vi "Z_ROI_compiler.vi"(0 "AOL_Globals":T2={"Imaging Protocol"=enum."AOL Z-Stack", "Number of POI"=0, "Number of Miniscans"=0, "Number of Trials"=0, "Number of Cycles "=0, "# Averaged Frames"=0, "Laser power (%)"=0, "Pockels (V)"=0.0, "Acquisition Length (sec)"=0.0, "Fill time (us)"=0.0, "POI Dwell time (us)"=0.0, "Miniscan Dwell time per pixel (us)"=0.0, "PMT 1"=0.0, "PMT 2"=0.0, "Back Apperture (mA)"=200.0, "Frame Size"=0, "Center Frequency"=0.0, "Field of View (um)"=175.0, "Field of View (norm)"=0.0, "DwellTime (us)"=0.0, "Ref Dwell Time (us)"=0.0, "Wavelength (nm)"=0.0, "Zoom"=0.0, "AOL Z"=0.0, "AOL Mode"=enum."Raster", "GridXY"=0.0, "GridZ"=0.0, "TriggerPeriod (sec)"=0.0, "Number of Pixels in Miniscan"=0, "Experiment folder path"=path "", "X centre"=0.0, "Y centre"=0.0, "Angle (degrees)"=0.0, "Angle Xs (degrees)"=0.0, "Angle Ys (degrees)"=0.0, "Plane Mode"=0, "Threshold"=[], "Regenerate Chirps"=FALSE, "Rectangle ROI length (pixels)"=0, "Rectangle ROI height (pixels)"=0, "AOD fill"=4900, "StartupDelay"=0, "Samples Wait after Trigger"=5080, "Slip Cycle"=600000, "Add Cycle"=TRUE, "Functional Mode"=enum."Point", "Z Start"=0.0, "Z Stop"=0.0, "# Planes"=0, "Total Pixels"=0, "Variable Miniscan Pixels"=[], "Use Variable Length"=FALSE, "Use Variable Resolution"=FALSE, "Laser power (%) at Z Start"=0, "Laser power (%) at Z Stop"=0, "Ref Z Step"=0} {"Angle Ys (degrees)" format="%#.6g"; "Angle Xs (degrees)" format="%#.6g"; "Plane Mode" items=["XY Plane", "XZ Plane", "YZ Plane", "arbitraryplane"]; "Frame Size" items=["100X100"=100, "128X128"=128, "200X200"=200, "256X256"=256, "512X512"=512, "1024x1024"=1024, "2048x2048"=2048]; "Back Apperture (mA)" format="%#.6g"; "Pockels (V)" format="%#.6g"; "PMT 2" format="%#.6g"; "PMT 1" format="%#.6g"; "Angle (degrees)" format="%#.6g"; "POI Dwell time (us)" format="%#.6g"}, 1 "dISABLE":bool=TRUE, 5 "Acquired z-plane index / volume index":i32, 11 "error in (no error)":errorcluster) -> (2 "Laser(V)":dbl[](array[numeric]), 3 "Zoom":dbl[](array[numeric]), 4 "Cycle time (us)":dbl, 6 "ROI Coordinates (broken down to miniscans)":T8, 10 "AOL_Globals":T2={"Imaging Protocol"=enum."AOL Z-Stack", "Number of POI"=0, "Number of Miniscans"=0, "Number of Trials"=0, "Number of Cycles "=0, "# Averaged Frames"=0, "Laser power (%)"=0, "Pockels (V)"=0.0, "Acquisition Length (sec)"=0.0, "Fill time (us)"=0.0, "POI Dwell time (us)"=0.0, "Miniscan Dwell time per pixel (us)"=0.0, "PMT 1"=0.0, "PMT 2"=0.0, "Back Apperture (mA)"=200.0, "Frame Size"=0, "Center Frequency"=0.0, "Field of View (um)"=175.0, "Field of View (norm)"=0.0, "DwellTime (us)"=0.0, "Ref Dwell Time (us)"=0.0, "Wavelength (nm)"=0.0, "Zoom"=0.0, "AOL Z"=0.0, "AOL Mode"=enum."Raster", "GridXY"=0.0, "GridZ"=0.0, "TriggerPeriod (sec)"=0.0, "Number of Pixels in Miniscan"=0, "Experiment folder path"=path "", "X centre"=0.0, "Y centre"=0.0, "Angle (degrees)"=0.0, "Angle Xs (degrees)"=0.0, "Angle Ys (degrees)"=0.0, "Plane Mode"=0, "Threshold"=[], "Regenerate Chirps"=FALSE, "Rectangle ROI length (pixels)"=0, "Rectangle ROI height (pixels)"=0, "AOD fill"=4900, "StartupDelay"=0, "Samples Wait after Trigger"=5080, "Slip Cycle"=600000, "Add Cycle"=TRUE, "Functional Mode"=enum."Point", "Z Start"=0.0, "Z Stop"=0.0, "# Planes"=0, "Total Pixels"=0, "Variable Miniscan Pixels"=[], "Use Variable Length"=FALSE, "Use Variable Resolution"=FALSE, "Laser power (%) at Z Start"=0, "Laser power (%) at Z Stop"=0, "Ref Z Step"=0} {"Angle Ys (degrees)" format="%#.6g"; "Angle Xs (degrees)" format="%#.6g"; "Plane Mode" items=["XY Plane", "XZ Plane", "YZ Plane", "arbitraryplane"]; "Frame Size" items=["100X100"=100, "128X128"=128, "200X200"=200, "256X256"=256, "512X512"=512, "1024x1024"=1024, "2048x2048"=2048]; "Back Apperture (mA)" format="%#.6g"; "Pockels (V)" format="%#.6g"; "PMT 2" format="%#.6g"; "PMT 1" format="%#.6g"; "Angle (degrees)" format="%#.6g"; "POI Dwell time (us)" format="%#.6g"}, 12 "NO ROI AVAILABLE!!!":bool, 13 "ROI Attributes (broken down to miniscans)":T1[](array[typedef]) {"Apparent Frame Size" format="%#_6f"; "Original FOV (um)" format="%#_6f"; "Pixels per miniscan" format="%#_6f"; "Dwell Time per pixel" format="%#_6f"; "Resolution" format="%#_6f"; "ROI group ID" format="%#_6f"; "Laser Power (%)" format="%#_6f"; "Zoom" format="%#_6f"; "Frame Size" format="%#_6f"; "Number of lines" format="%#_6f"; "Composite ID" format="%#_6f"; "Angle (deg)" format="%#_6f"; "ROI Time (ns)" format="%#_6f"; "ROI ID" format="%#_6f"; "Pixels in ROI" format="%#_6f"; "ROI index" format="%#_6f"; "Z stop" format="%#_6f"; "Y stop" format="%#_6f"; "X stop" format="%#_6f"; "Z start" format="%#_6f"; "X start" format="%#_6f"; "Y start" format="%#_6f"}, 15 "error out":errorcluster)   [LabVIEW 2020]
uses:
  Typedefs/ROI XY coordinates cluster.ctl
  Typedefs/Controls/AOL_Globals.ctl
  Typedefs/Imaging Protocols enum.ctl
  Typedefs/Frame Size.ctl
  Typedefs/AOL modes.ctl
  Typedefs/Plane Mode.ctl
  Typedefs/Functional Mode.ctl
  User Interface/Visualisation/Functional Imaging Viewer/Typedefs/ROI parameters data type.ctl
  User Interface/Visualisation/Functional Imaging Viewer/SubVIs/Experiment header interface/Typedefs/Header file sections.ctl
  User Interface/Visualisation/Functional Imaging Viewer/SubVIs/Experiment header interface/Typedefs/Header file actions.ctl
  User Interface/Visualisation/Functional Imaging Viewer/SubVIs/Experiment header interface/Typedefs/Save-Load-Save as-Load last enum.ctl
  User Interface/Visualisation/Functional Imaging Viewer/SubVIs/Experiment header interface/Typedefs/Header file type enum.ctl
panel:
  # "PRE-ALLOCATED CLONE RE-ENTRANT"
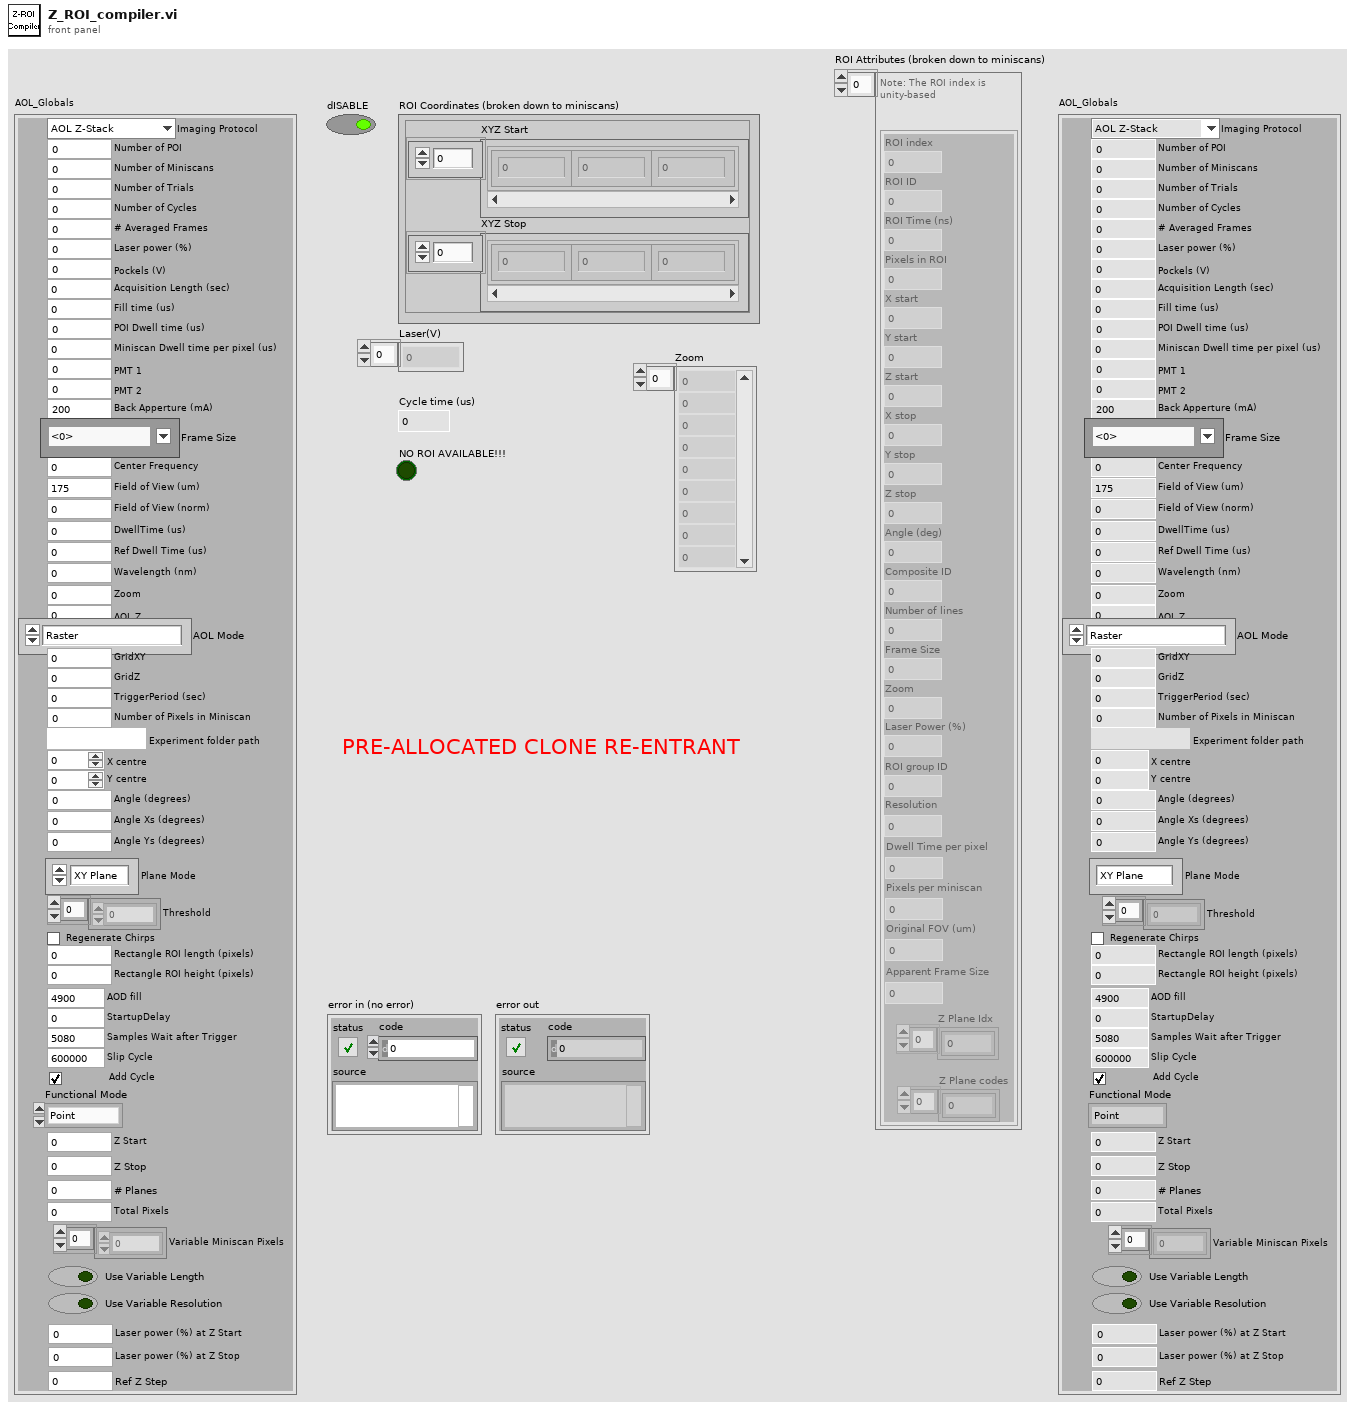
[diagram p1: front panel]
types:
  T1 = typedef "ROI parameters data type.ctl" = cluster{"ROI index":dbl, "ROI ID":dbl, "ROI Time (ns)":dbl, "Pixels in ROI":dbl, "X start":dbl, "Y start":dbl, "Z start":dbl, "X stop":dbl, "Y stop":dbl, "Z stop":dbl, "Angle (deg)":dbl, "Composite ID":dbl, "Number of lines":dbl, "Frame Size":dbl, "Zoom":dbl, "Laser Power (%)":dbl, "ROI group ID":dbl, "Resolution":dbl, "Dwell Time per pixel":dbl, "Pixels per miniscan":dbl, "Original FOV (um)":dbl, "Apparent Frame Size":dbl, "Z Plane Idx":i32[], "Z Plane codes":i32[]}
  T2 = typedef "AOL_Globals.ctl" = cluster{"Imaging Protocol":T3, "Number of POI":u16, "Number of Miniscans":u16, "Number of Trials":u16, "Number of Cycles ":u64, "# Averaged Frames":u16, "Laser power (%)":u8, "Pockels (V)":dbl, "Acquisition Length (sec)":dbl, "Fill time (us)":dbl, "POI Dwell time (us)":dbl, "Miniscan Dwell time per pixel (us)":dbl, "PMT 1":dbl, "PMT 2":dbl, "Back Apperture (mA)":dbl, "Frame Size":T4, "Center Frequency":dbl, "Field of View (um)":dbl, "Field of View (norm)":dbl, "DwellTime (us)":dbl, "Ref Dwell Time (us)":dbl, "Wavelength (nm)":dbl, "Zoom":dbl, "AOL Z":dbl, "AOL Mode":T5, "GridXY":dbl, "GridZ":dbl, "TriggerPeriod (sec)":dbl, "Number of Pixels in Miniscan":u16, "Experiment folder path":path, "X centre":dbl, "Y centre":dbl, "Angle (degrees)":dbl, "Angle Xs (degrees)":dbl, "Angle Ys (degrees)":dbl, "Plane Mode":T6, "Threshold":u16[], "Regenerate Chirps":bool, "Rectangle ROI length (pixels)":u16, "Rectangle ROI height (pixels)":u16, "AOD fill":u16, "StartupDelay":i32, "Samples Wait after Trigger":u16, "Slip Cycle":u32, "Add Cycle":bool, "Functional Mode":T7, "Z Start":dbl, "Z Stop":dbl, "# Planes":i32, "Total Pixels":i32, "Variable Miniscan Pixels":u16[], "Use Variable Length":bool, "Use Variable Resolution":bool, "Laser power (%) at Z Start":u8, "Laser power (%) at Z Stop":u8, "Ref Z Step":i8}
  T3 = typedef "Imaging Protocols enum.ctl" = enum16{"AOL Z-Stack", "Motor Z Stack", "Parameter Sweep", "Functional Acquisition", "Single Plane Acquisition", "Volume Acquisition", "Live Imaging", "Live Plane Imaging", "Live Volume Imaging"}
  T4 = typedef "Frame Size.ctl" = u16
  T5 = typedef "AOL modes.ctl" = enum16{"Raster", "Structural", "Pointing", "Mini Scan", "Alignment"}
  T6 = typedef "Plane Mode.ctl" = u16
  T7 = typedef "Functional Mode.ctl" = enum16{"Point", "Line", "Patch", "Plane", "Volume"}
  T8 = typedef "ROI XY coordinates cluster.ctl" = cluster{"XYZ Start":cluster{"X":sgl, "Y":sgl, "Z":sgl}[], "XYZ Stop":cluster{"X":sgl, "Y":sgl, "Z":sgl}[]}
  T9 = typedef "Header file actions.ctl" = enum16{"Create", "Open", "Read All", "Read Section", "Write All", "Write Section", "Close"}
  T10 = typedef "Header file sections.ctl" = enum16{"ALL SECTIONS", "LOGIN", "GLOBAL PARAMETERS", "CALIBRATION DATA", "IMAGING MODES", "TIME SERIES", "MOTOR Z-STACK", "AOL Z-STACK", "FUNCTIONAL IMAGING", "VOLUME IMAGING", "MOVEMENT CORRECTION", "CALIBRATION", "STATISTICS", "BIOLOGY INFORMATION"}
  T11 = typedef "Header file type enum.ctl" = enum16{"All parameters", "Params for funct acq w ROI or mscn", "Params for funct acq w rectangles", "Live imaging header parameters", "AOL Parameters"}
  T12 = typedef "Save-Load-Save as-Load last enum.ctl" = enum16{"Save file", "Save file as", "Load file", "Load last file"}
  T13 = typedef "Header parameters cluster-ALL.ctl" = cluster{"LOGIN":T14, "GLOBAL PARAMETERS":T15, "IMAGING MODES":T17, "TIME SERIES":T18, "MOTOR Z-STACK ":T20, "AOL Z-STACK":T21, "FUNCTIONAL IMAGING":T22, "VOLUME IMAGING":T22, "MOVEMENT CORRECTION":T23, "CALIBRATION":T25, "STATISTICS":T26, "BIOLOGY INFORMATION":T27, "Calibration Data":T28}
  T14 = typedef "Header params -Login.ctl" = cluster{"User":string, "Profile":string, "Software Version":string, "Experiment Date Time":timestamp}
  T15 = typedef "Header params-Global Parameters.ctl" = cluster{"MicroscopeID":string, "Microscope Type":string, "Objective":string, "Field of View (um)":dbl, "Fill time (us)":dbl, "Experiment Type":T16, "Stimuli Trigger":bool, "Speed Logging":bool}
  T16 = typedef "Experiment Type.ctl" = enum16{"In vivo", "In vitro", "Testing", "Calibration", "Other"}
  T17 = typedef "Header params-Imaging Modes.ctl" = cluster{"Time Series":bool, "Motor Zstack":bool, "AOL Zstack":bool, "Functional Imaging":bool, "Volume Imaging":bool}
  T18 = typedef "Header params-Time Series.ctl" = cluster{"Basic Image meta data":T19, "AOL z":dbl}
  T19 = typedef "Header params-Basic image meta data.ctl" = cluster{"Wavelength (nm)":dbl, "# averaged frames":dbl, "laser power (%)":dbl, "Pockels":dbl, "pixel dwell time (us)":dbl, "pmt 1":dbl, "pmt 2":dbl, "back apperture":dbl, "zoom":dbl, "field of view":dbl, "Frame Size":T4, "AOL x centre":dbl, "AOL y centre":dbl, "Stage x position":dbl, "Stage y position":dbl, "Stage z position":dbl}
  T20 = typedef "Header params-Motor Z-stack.ctl" = cluster{"Hdr Basic Image meta data":T19, "Z Start":dbl, "Z Stop":dbl, "No of Planes":i32, "Laser Power (%) at Z Start":dbl, "Laser Power (%) at Z Stop":dbl}
  T21 = typedef "Header params-AOL Z-stack.ctl" = cluster{"Hdr Basic Image meta data":T19, "Z Start":dbl, "Z Stop":dbl, "No of Planes":i32, "Laser Power (%) at Z Start":dbl, "Laser Power (%) at Z Stop":dbl}
  T22 = typedef "Header params-Functional Imaging.ctl" = cluster{"Functional Mode":T7, "Variable Length":bool, "Variable Resolution":bool, "Pockels Modulation":bool, "Stimuli Trigger":bool, "Cool down enabled":bool, "AOL Mode":T5, "Plane Mode":T6, "Miniscan Dwell time per pixel (us)":dbl, "poi dwell time":dbl, "Number of trials":dbl, "Number of cycles":dbl, "Number of pois":dbl, "Number of miniscans":dbl, "Number of pixels in miniscan":dbl, "Rectangle ROI length":dbl, "Rectangle ROI height":dbl, "Frame rate (fps)":dbl, "Acquisition Length":dbl, "video length (sec)":dbl, "Stimuli delay (sec)":dbl, "Cool down time (sec)":dbl, "Basic Image meta data":T19, "Z Start (um)":dbl, "Z Stop (um)":dbl}
  T23 = typedef "Header params-Movement correction.ctl" = cluster{"Movement Correction":bool, "Axial Reference":bool, "Reference Source":T24, "Full Frame Size":dbl, "Reference Field of View":dbl, "Reference Zoom":dbl, "Reference dwell time (us)":dbl, "Reference X Pixels":dbl, "Reference Y Pixels":dbl, "Number of Z lines":dbl, "Size of Z pixels":dbl, "Axial Pixels":dbl, "Ignore Z lines":dbl, "Reference Scan Cycles":dbl, "Reference Threshold XY":dbl, "Reference Threshold Z":dbl, "Reference Average XY":dbl, "Reference Average Z":dbl, "Proportional Scale":dbl, "Integral Scale":dbl, "Proportional Scale Z":dbl, "Integral Scale Z":dbl, "Diff Threshold":dbl, "Diff Threshold Z":dbl, "Sliding Average":bool, "Reference count reset enabled":bool, "Scan Interval (ms)":dbl, "Ref Plot Refresh Rate (ms)":dbl}
  T24 = typedef "Reference source.ctl" = enum16{"Green channel", "Red channel"}
  T25 = typedef "Header params-Calibration Setup.ctl" = cluster{"Pockels Calibration File":path, "Calibration_ini file":path, "Setup_ini file":path}
  T26 = typedef "Header params-statistics.ctl" = cluster{"Z-stack duration (sec)":dbl, "Number of acquired data-points":dbl, "Acquisition time (ms)":dbl, "Number of acquired frames":dbl, "Intertrial times":dbl[]}
  T27 = typedef "Biology Information.ctl" = cluster{"Animal Code or Name":string, "Animal DoB":string, "Animal Age":string, "Animal Sex":string, "Animal Weight":string, "Date of Injection":string, "Date of Implant":string, "Site of Injection":string, "Animal Ear Notch":string, "AAV constructs":string, "Genetic background":string, "Optical reporter":string, "Region of brain imaged":string, "Other \ncomments":string}
  T28 = typedef "Header params-calibration data.ctl" = cluster{"Objective Name":string, "Calibration Wavelength":dbl, "Sum X":dbl, "Sum Y":dbl, "Diff X":dbl, "Diff Y":dbl, "Distortion Correction":dbl, " Z norm to um Scaling":dbl, " X norm to um Scaling":dbl}
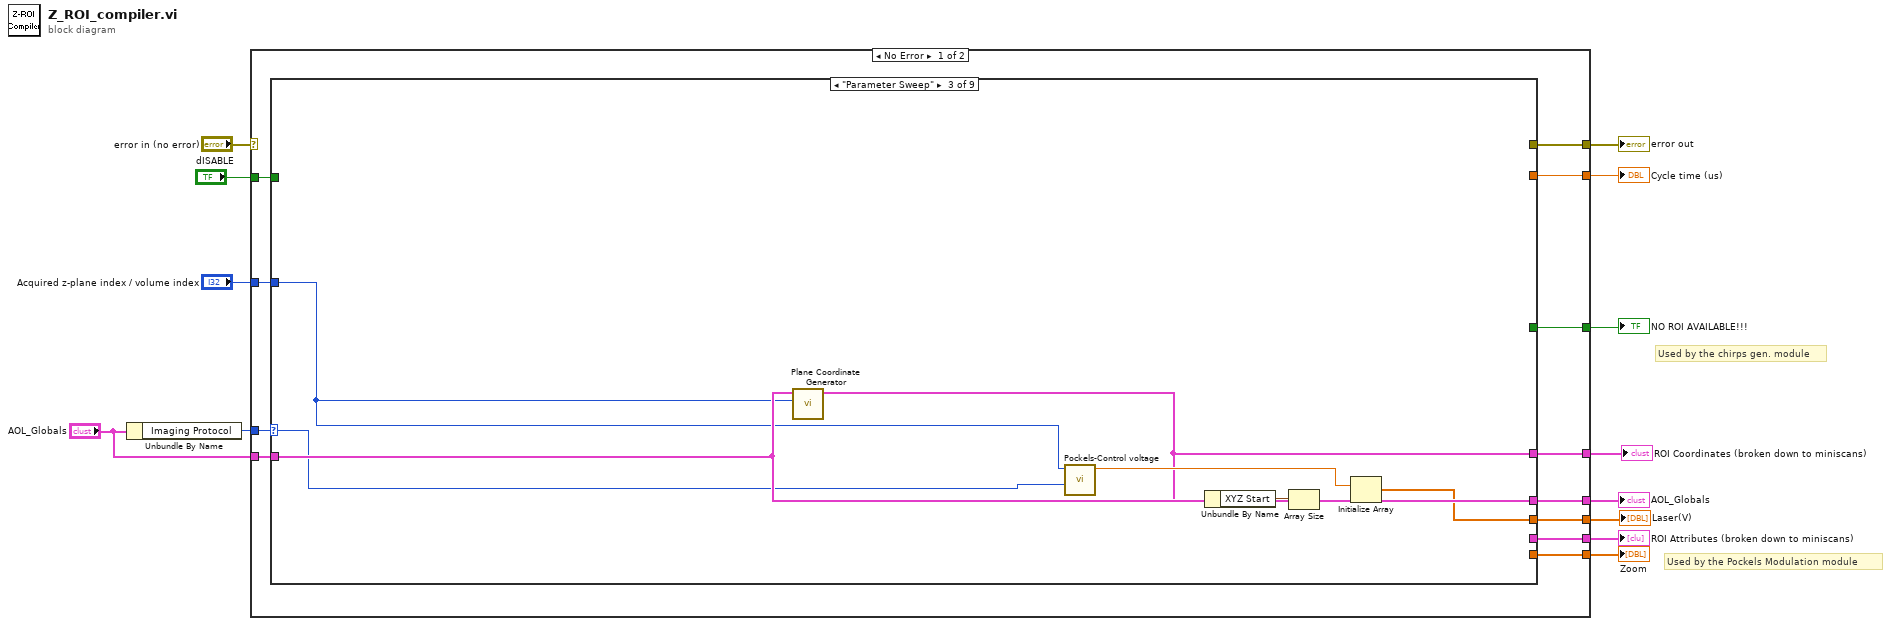
[diagram p0: block diagram]
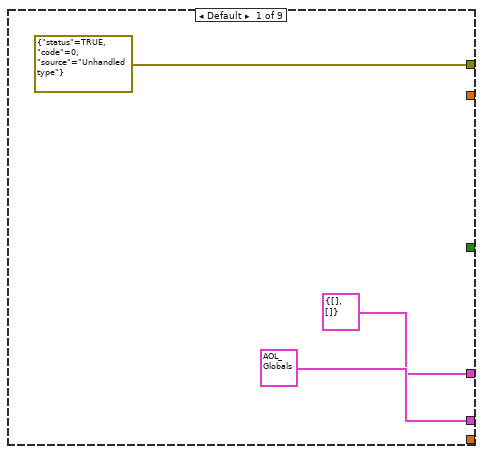
[diagram p2: hidden frame]
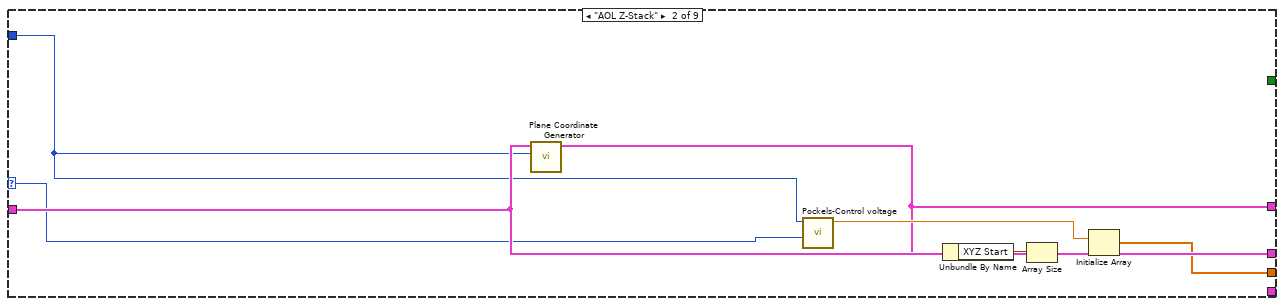
[diagram p3: hidden frame]
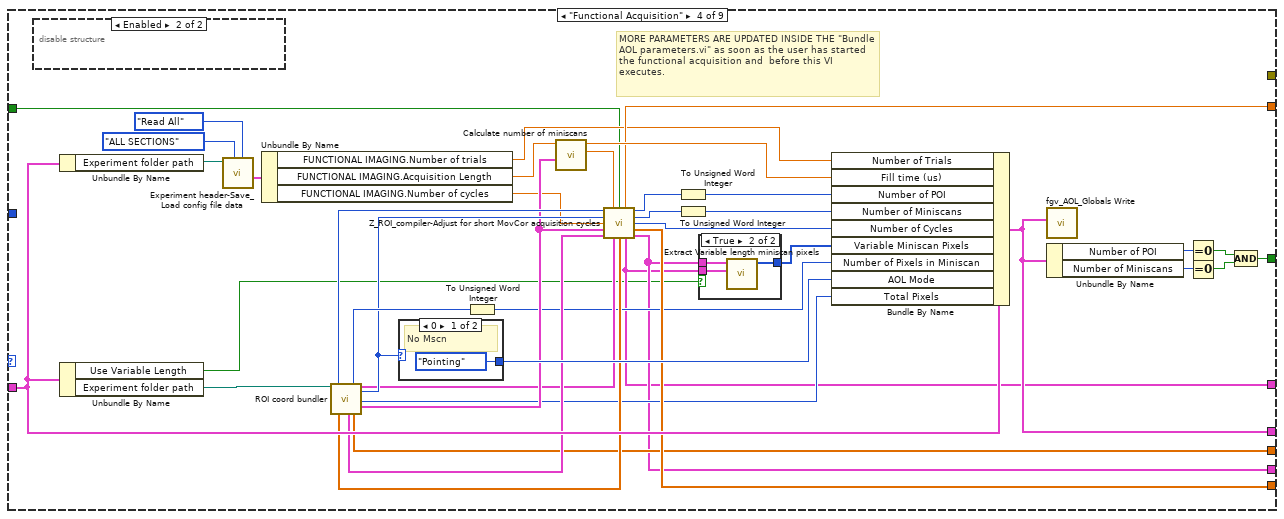
[diagram p4: hidden frame]
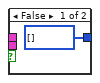
[diagram p5: hidden frame]
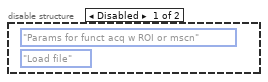
[diagram p6: hidden frame]
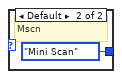
[diagram p7: hidden frame]
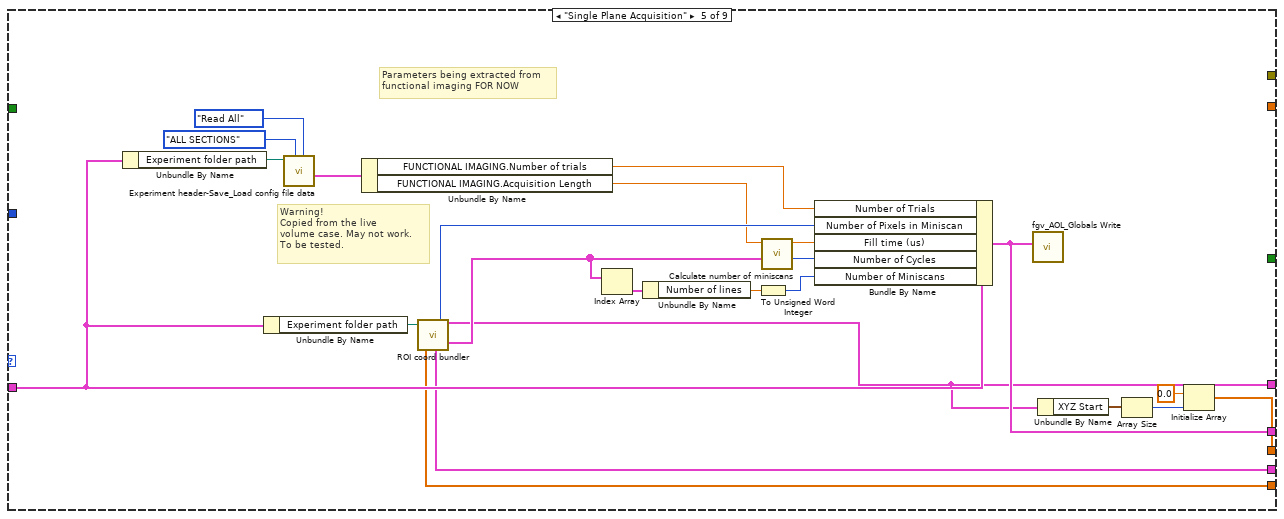
[diagram p8: hidden frame]
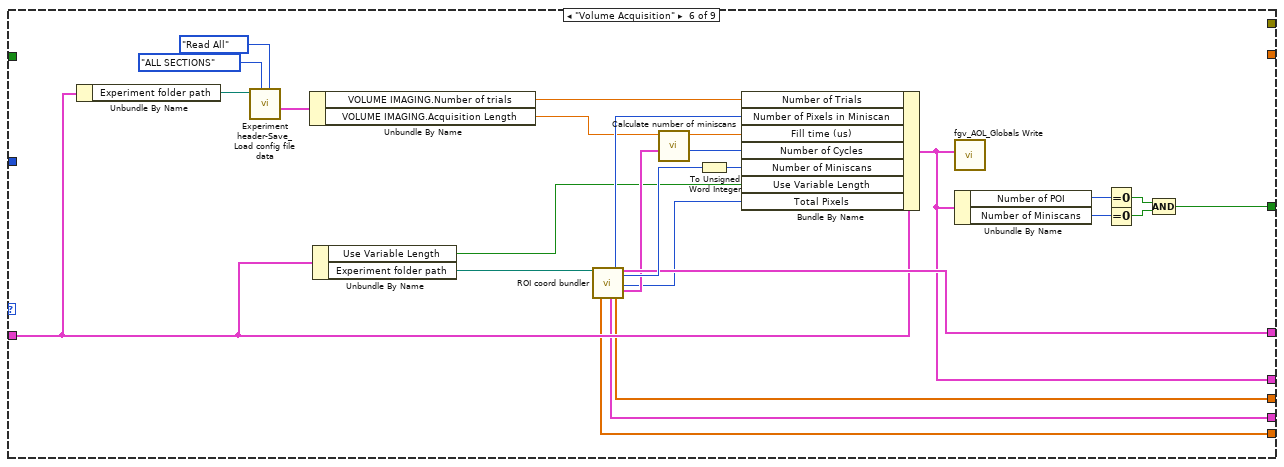
[diagram p9: hidden frame]
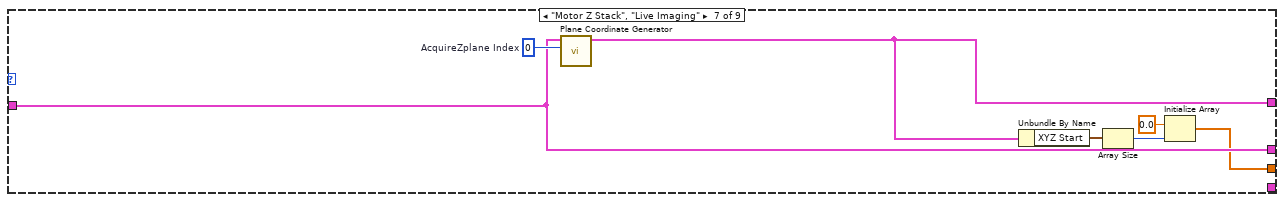
[diagram p10: hidden frame]
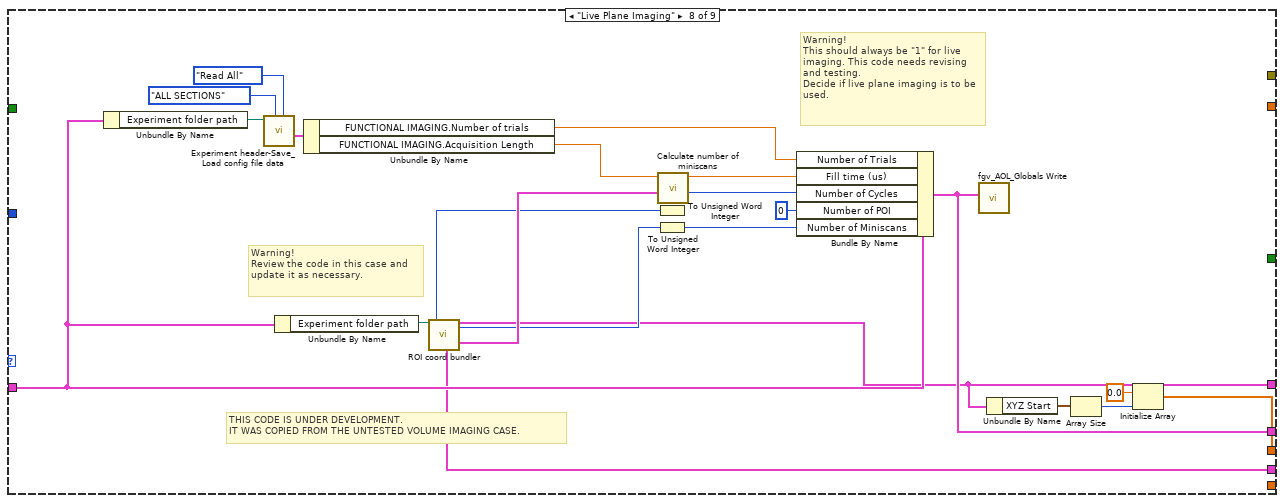
[diagram p11: hidden frame]
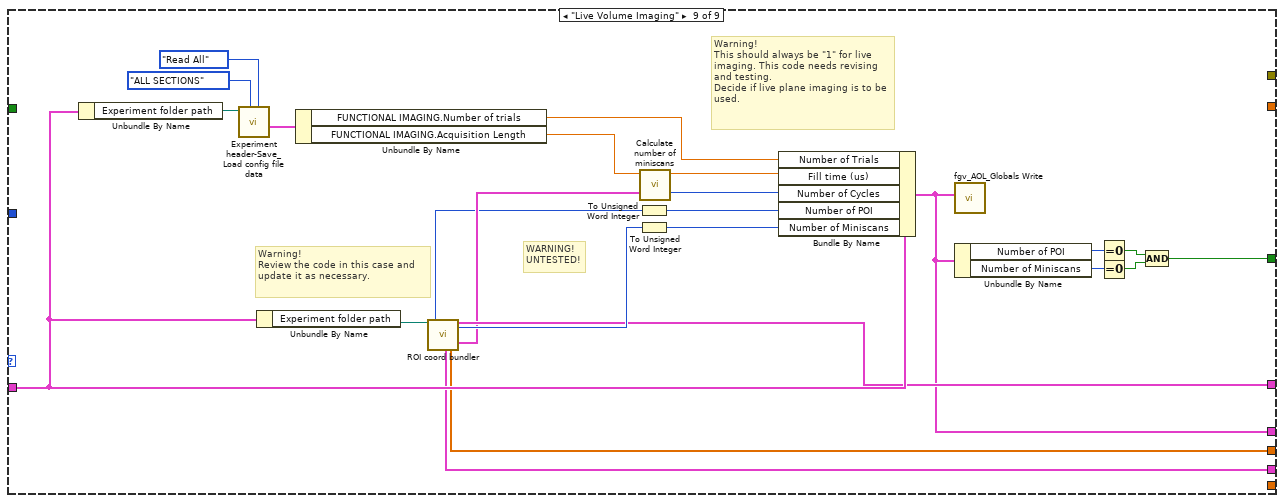
[diagram p12: hidden frame]
diagram:
  # "Used by the Pockels Modulation module"
  # "Used by the chirps gen. module"
  n1 = Unbundle By Name("AOL_Globals") -> ("Imaging Protocol"=w11:T3)
  n2 = case shown="No Error" "error in (no error)" {
    selector: "error in (no error)" -> [_ w193]
    tunnel: "Acquired z-plane index / volume index" -> [w25 _]
    tunnel: [w24 _] -> w12
    tunnel: w11 -> [w23 _]
    tunnel: [w22 w193] -> w10
    tunnel: "AOL_Globals" -> [w21 _]
    tunnel: [w20 _] -> w4
    tunnel: [w19 _] -> w7
    tunnel: [w18 _] -> w6
    tunnel: [w17 _] -> w5
    tunnel: [w16 _] -> w3
    tunnel: "dISABLE" -> [w15 _]
    tunnel: [w14 _] -> w1
    frame No Error {
      n3 = case shown="\"Parameter Sweep\"" w23 {
        selector: w23 -> [_ w35 w43 _ _ _ _ _ _]
        tunnel: [T8 {"XYZ Start"=[], "XYZ Stop"=[]} ("miniScan_Coordinates") w29 w37 w46 w95 w134 w144 w151 w182] -> w24
        tunnel: w25 -> [_ w34 w42 _ _ _ _ _ _]
        tunnel: w21 -> [_ w36 w44 w79 w101 w121 w145 w162 w185]
        tunnel: [errorcluster {"status"=TRUE, "code"=0, "source"="Unhandled type"} ("error out") _ _ _ _ _ _ _ _] -> w22
        tunnel: [T2 {"Imaging Protocol"=enum."AOL Z-Stack", "Number of POI"=0, "Number of Miniscans"=0, "Number of Trials"=0, "Number of Cycles "=0, "# Averaged Frames"=0, "Laser power (%)"=0, "Pockels (V)"=0.0, "Acquisition Length (sec)"=0.0, "Fill time (us)"=0.0, "POI Dwell time (us)"=0.0, "Miniscan Dwell time per pixel (us)"=0.0, "PMT 1"=0.0, "PMT 2"=0.0, "Back Apperture (mA)"=200.0, "Frame Size"=0, "Center Frequency"=0.0, "Field of View (um)"=175.0, "Field of View (norm)"=0.0, "DwellTime (us)"=0.0, "Ref Dwell Time (us)"=0.0, "Wavelength (nm)"=0.0, "Zoom"=0.0, "AOL Z"=0.0, "AOL Mode"=enum."Raster", "GridXY"=0.0, "GridZ"=0.0, "TriggerPeriod (sec)"=0.0, "Number of Pixels in Miniscan"=0, "Experiment folder path"=path "", "X centre"=0.0, "Y centre"=0.0, "Angle (degrees)"=0.0, "Angle Xs (degrees)"=0.0, "Angle Ys (degrees)"=0.0, "Plane Mode"=0, "Threshold"=[], "Regenerate Chirps"=FALSE, "Rectangle ROI length (pixels)"=0, "Rectangle ROI height (pixels)"=0, "AOD fill"=0, "StartupDelay"=0, "Samples Wait after Trigger"=0, "Slip Cycle"=0, "Add Cycle"=FALSE, "Functional Mode"=enum."Point", "Z Start"=0.0, "Z Stop"=0.0, "# Planes"=0, "Total Pixels"=0, "Variable Miniscan Pixels"=[], "Use Variable Length"=FALSE, "Use Variable Resolution"=FALSE, "Laser power (%) at Z Start"=0, "Laser power (%) at Z Stop"=0, "Ref Z Step"=0} ("AOL_Globals") w36 w44 w70 w102 w123 w145 w160 w175] -> w20
        tunnel: [_ _ _ w63 _ _ _ _ _] -> w19
        tunnel: [_ _ _ w48 w98 w120 _ w155 w172] -> w18
        tunnel: [_ _ _ w57 w99 w119 _ _ _] -> w17
        tunnel: [_ _ _ w69 _ w122 _ _ w174] -> w16
        tunnel: w15 -> [_ _ _ w56 _ _ _ _ _]
        tunnel: [_ w31 w39 w53 w93 w118 w141 w149 w171] -> w14
        frame Default {
        }
        frame "AOL Z-Stack" {
          n4 = call "Plane Coordinate Generator.vi"("AcquireZplane Index"=w34, "AOL_Globals"=w36) -> ("ROI Attributes (broken down to miniscans)"=w29:T8)  [unwired: 8 in, 1 out]
          n5 = call "Pockels-Control voltage.vi"("Imaging Protocol"=w35, "Index of Z-plane"=w34) -> ("Pockels control voltage (V)"=w30:dbl)  [unwired: 8 in, 1 out]
          n6 = Unbundle By Name(w29) -> ("XYZ Start"=w33:cluster{"X":sgl, "Y":sgl, "Z":sgl}[])
          n7 = Array Size(array=w33) -> (size(s)=w32:i32)
          n8 = Initialize Array(w30, w32) -> (w31:dbl[])
        }
        frame "Parameter Sweep" {
          n9 = call "Plane Coordinate Generator.vi"("AcquireZplane Index"=w42, "AOL_Globals"=w44) -> ("ROI Attributes (broken down to miniscans)"=w37:T8)  [unwired: 8 in, 1 out]
          n10 = call "Pockels-Control voltage.vi"("Imaging Protocol"=w43, "Index of Z-plane"=w42) -> ("Pockels control voltage (V)"=w38:dbl)  [unwired: 8 in, 1 out]
          n11 = Unbundle By Name(w37) -> ("XYZ Start"=w41:cluster{"X":sgl, "Y":sgl, "Z":sgl}[])
          n12 = Array Size(array=w41) -> (size(s)=w40:i32)
          n13 = Initialize Array(w38, w40) -> (w39:dbl[])
        }
        frame "Functional Acquisition" {
          # "MORE PARAMETERS ARE UPDATED INSIDE THE \"Bundle AOL parameters.vi\" as soon as the user has started the functional acquisition and  before this VI executes."
          n14 = disable-structure shown="Enabled" {
            frame Disabled {
              (unwired) Header_file_type_enum."Params for funct acq w ROI or mscn" ("Header file type")
              (unwired) Save-Load-Save_as-Load_last_enum."Load file" ("Function")
            }
            frame Enabled {
            }
          }
          n15 = Unbundle By Name(w79) -> ("Experiment folder path"=w82:path)
          n16 = Unbundle By Name(w79) -> ("Use Variable Length"=w45:bool, "Experiment folder path"=w78:path)
          n17 = call "Experiment header-Save_Load config file data.vi"("Header file actions"=Header_file_actions."Read All", "Header file sections"=Header_file_sections."ALL SECTIONS", "Experiment data folder path"=w82) -> ("All header parameters out"=w81:T13)  [unwired: 7 in, 1 out]
          n18 = Unbundle By Name(w81) -> ("FUNCTIONAL IMAGING.Number of trials"=w60:dbl, "FUNCTIONAL IMAGING.Acquisition Length"=w80:dbl, "FUNCTIONAL IMAGING.Number of cycles"=w54:dbl)
          n19 = call "ROI coord bundler.vi"("Experiment folder path"=w78) -> ("Number of POIs"=w68:i32, "Zoom"=w58:dbl[], "ROI Attributes (broken down to miniscans)"=w61:T1[], "Number of pixels in single miniscan"=w77:i32, "Laser(V)"=w53:dbl[], "ROI Coordinates (broken down to miniscans)"=w59:T8, "Total number of miniscans"=w66:i32, "Total Pixels"=w50:i32, "ROI Attributes"=w62:T1[])  [unwired: 8 in, 2 out]
          n20 = case shown="0" w66 {
            tunnel: [AOL_modes."Pointing" ("AOL Mode") AOL_modes."Mini Scan" ("AOL Mode")] -> w75
            frame 0 {
              # "No Mscn"
            }
            frame Default {
              # "Mscn"
            }
          }
          n21 = To Unsigned Word Integer(number=w77) -> (unsigned 16bit integer=w49:u16)
          n22 = call "Calculate number of miniscans.vi"("XYZ Coordinates"=w62, "Acquisition length (sec)"=w80) -> ("Cycle time (us)"=w64:dbl, "AOD fill time (us)"=w84:dbl)  [unwired: 7 in, 1 out]
          n23 = call "Z_ROI_compiler-Adjust for short MovCor acquisition cycles.vi"("Number of POIs"=w68, "Cycle time (us)"=w64, "dISABLE"=w56, "Total number of miniscans"=w66, "Number of cycles"=w54, "ROI Attributes"=w62, "ROI Attributes (broken down to miniscans) in"=w61, "ROI Coordinates (broken down to miniscans) in"=w59, "Zoom"=w58) -> ("Cycle time (us) (multiplied by number of stacked cycles)"=w63:dbl, "Number of POIs (multiplied by number of stacked cycles)"=w67:i32, "Number of miniscans (multiplied by number of stacked cycles)"=w65:i32, "Number of cycles or number of stacked cycles"=w55:u64, "Zoom"=w57:dbl[], "ROI Coordinates (broken down to miniscans) out"=w46:T8, "ROI Attributes (broken down to miniscans) out"=w48:T1[])
          n24 = To Unsigned Word Integer(number=w67) -> (unsigned 16bit integer=w83:u16)
          n25 = To Unsigned Word Integer(number=w65) -> (unsigned 16bit integer=w76:u16)
          n26 = case shown="True" w45 {
            tunnel: w48 -> [_ w88]
            tunnel: [u16[] [] ("Pixels per miniscan") w87] -> w47
            tunnel: w46 -> [_ w86]
            frame False {
            }
            frame True {
              n27 = call "Extract Variable length miniscan pixels.vi"("ROI Coordinates (broken down to miniscans) out"=w86, "ROI Attributes (broken down to miniscans)"=w88) -> ("Pixels per miniscan"=w87:u16[])  [unwired: 8 in, 1 out]
            }
          }
          n28 = Bundle By Name(cluster=w79, "Number of Trials"=w60, "Fill time (us)"=w84, "Number of POI"=w83, "Number of Miniscans"=w76, "Number of Cycles"=w55, "Variable Miniscan Pixels"=w47, "Number of Pixels in Miniscan"=w49, "AOL Mode"=w75, "Total Pixels"=w50) -> (w70:T2)
          n29 = call "fgv_AOL_Globals Write.vi"("AOL_Globals"=w70) -> ()  [unwired: 10 in, 1 out]
          n30 = Unbundle By Name(w70) -> ("Number of POI"=w73:u16, "Number of Miniscans"=w74:u16)
          n31 = Equal To 0?(x=w73) -> (x = 0?=w72:bool)
          n32 = Equal To 0?(x=w74) -> (x = 0?=w71:bool)
          n33 = Compound Arithmetic op=AND(w72, w71) -> (w69:bool)
        }
        frame "Single Plane Acquisition" {
          # "Parameters being extracted from\nfunctional imaging FOR NOW"
          # "Warning!\nCopied from the live\nvolume case. May not work.\nTo be tested."
          n34 = Unbundle By Name(w101) -> ("Experiment folder path"=w108:path)
          n35 = Unbundle By Name(w101) -> ("Experiment folder path"=w110:path)
          n36 = call "Experiment header-Save_Load config file data.vi"("Header file actions"=Header_file_actions."Read All", "Header file sections"=Header_file_sections."ALL SECTIONS", "Experiment data folder path"=w108) -> ("All header parameters out"=w107:T13)  [unwired: 7 in, 1 out]
          n37 = Unbundle By Name(w107) -> ("FUNCTIONAL IMAGING.Number of trials"=w105:dbl, "FUNCTIONAL IMAGING.Acquisition Length"=w106:dbl)
          n38 = call "ROI coord bundler.vi"("Experiment folder path"=w110) -> ("Zoom"=w99:dbl[], "ROI Attributes (broken down to miniscans)"=w98:T1[], "Number of pixels in single miniscan"=w109:i32, "ROI Coordinates (broken down to miniscans)"=w95:T8, "ROI Attributes"=w100:T1[])  [unwired: 8 in, 6 out]
          n39 = Index Array(array=w100) -> (element=w104:T1)  [unwired: 1 in]
          n40 = Unbundle By Name(w104) -> ("Number of lines"=w103:dbl)
          n41 = To Unsigned Word Integer(number=w103) -> (unsigned 16bit integer=w112:u16)
          n42 = call "Calculate number of miniscans.vi"("XYZ Coordinates"=w100, "Acquisition length (sec)"=w106) -> ("Number of cycles"=w111:u64, "AOD fill time (us)"=w113:dbl)  [unwired: 7 in, 1 out]
          n43 = Bundle By Name(cluster=w101, "Number of Trials"=w105, "Number of Pixels in Miniscan"=w109, "Fill time (us)"=w113, "Number of Cycles"=w111, "Number of Miniscans"=w112) -> (w102:T2)
          n44 = call "fgv_AOL_Globals Write.vi"("AOL_Globals"=w102) -> ()  [unwired: 10 in, 1 out]
          n45 = Unbundle By Name(w95) -> ("XYZ Start"=w97:cluster{"X":sgl, "Y":sgl, "Z":sgl}[])
          n46 = Array Size(array=w97) -> (size(s)=w96:i32)
          n47 = Initialize Array(0.0 ("element"), w96) -> (w93:dbl[])
        }
        frame "Volume Acquisition" {
          n48 = Unbundle By Name(w121) -> ("Experiment folder path"=w132:path)
          n49 = call "Experiment header-Save_Load config file data.vi"("Header file actions"=Header_file_actions."Read All", "Header file sections"=Header_file_sections."ALL SECTIONS", "Experiment data folder path"=w132) -> ("All header parameters out"=w131:T13)  [unwired: 7 in, 1 out]
          n50 = Unbundle By Name(w131) -> ("VOLUME IMAGING.Number of trials"=w129:dbl, "VOLUME IMAGING.Acquisition Length"=w130:dbl)
          n51 = Unbundle By Name(w121) -> ("Use Variable Length"=w114:bool, "Experiment folder path"=w136:path)
          n52 = call "ROI coord bundler.vi"("Experiment folder path"=w136) -> ("Zoom"=w119:dbl[], "ROI Attributes (broken down to miniscans)"=w120:T1[], "Number of pixels in single miniscan"=w133:i32, "Laser(V)"=w118:dbl[], "ROI Coordinates (broken down to miniscans)"=w134:T8, "Total number of miniscans"=w135:i32, "Total Pixels"=w115:i32, "ROI Attributes"=w128:T1[])  [unwired: 8 in, 3 out]
          n53 = call "Calculate number of miniscans.vi"("XYZ Coordinates"=w128, "Acquisition length (sec)"=w130) -> ("Number of cycles"=w137:u64, "AOD fill time (us)"=w139:dbl)  [unwired: 7 in, 1 out]
          n54 = To Unsigned Word Integer(number=w135) -> (unsigned 16bit integer=w138:u16)
          n55 = Bundle By Name(cluster=w121, "Number of Trials"=w129, "Number of Pixels in Miniscan"=w133, "Fill time (us)"=w139, "Number of Cycles"=w137, "Number of Miniscans"=w138, "Use Variable Length"=w114, "Total Pixels"=w115) -> (w123:T2)
          n56 = call "fgv_AOL_Globals Write.vi"("AOL_Globals"=w123) -> ()  [unwired: 10 in, 1 out]
          n57 = Unbundle By Name(w123) -> ("Number of POI"=w126:u16, "Number of Miniscans"=w127:u16)
          n58 = Equal To 0?(x=w126) -> (x = 0?=w125:bool)
          n59 = Equal To 0?(x=w127) -> (x = 0?=w124:bool)
          n60 = Compound Arithmetic op=AND(w125, w124) -> (w122:bool)
        }
        frame "Motor Z Stack", "Live Imaging" {
          w146 = 0  # AcquireZplane Index
          n61 = call "Plane Coordinate Generator.vi"("AcquireZplane Index"=w146, "AOL_Globals"=w145) -> ("ROI Attributes (broken down to miniscans)"=w144:T8)  [unwired: 8 in, 1 out]
          n62 = Unbundle By Name(w144) -> ("XYZ Start"=w143:cluster{"X":sgl, "Y":sgl, "Z":sgl}[])
          n63 = Array Size(array=w143) -> (size(s)=w142:i32)
          n64 = Initialize Array(0.0 ("element"), w142) -> (w141:dbl[])
        }
        frame "Live Plane Imaging" {
          # "Warning!\nThis should always be \"1\" for live imaging. This code needs revising and testing.\nDecide if live plane imaging is to be used."
          # "THIS CODE IS UNDER DEVELOPMENT.\nIT WAS COPIED FROM THE UNTESTED VOLUME IMAGING CASE."
          # "Warning!\nReview the code in this case and update it as necessary."
          n65 = Unbundle By Name(w162) -> ("Experiment folder path"=w165:path)
          n66 = call "Experiment header-Save_Load config file data.vi"("Header file actions"=Header_file_actions."Read All", "Header file sections"=Header_file_sections."ALL SECTIONS", "Experiment data folder path"=w165) -> ("All header parameters out"=w164:T13)  [unwired: 7 in, 1 out]
          n67 = Unbundle By Name(w162) -> ("Experiment folder path"=w158:path)
          n68 = Unbundle By Name(w164) -> ("FUNCTIONAL IMAGING.Number of trials"=w161:dbl, "FUNCTIONAL IMAGING.Acquisition Length"=w163:dbl)
          n69 = call "ROI coord bundler.vi"("Experiment folder path"=w158) -> ("Number of POIs"=w156:i32, "ROI Attributes (broken down to miniscans)"=w155:T1[], "ROI Coordinates (broken down to miniscans)"=w151:T8, "Total number of miniscans"=w157:i32, "ROI Attributes"=w159:T1[])  [unwired: 8 in, 6 out]
          n70 = To Unsigned Word Integer(number=w156) -> ()  [unwired: 1 out]
          n71 = To Unsigned Word Integer(number=w157) -> (unsigned 16bit integer=w167:u16)
          n72 = call "Calculate number of miniscans.vi"("XYZ Coordinates"=w159, "Acquisition length (sec)"=w163) -> ("Number of cycles"=w166:u64, "AOD fill time (us)"=w168:dbl)  [unwired: 7 in, 1 out]
          n73 = Bundle By Name(cluster=w162, "Number of Trials"=w161, "Fill time (us)"=w168, "Number of Cycles"=w166, "Number of POI"=u16 0, "Number of Miniscans"=w167) -> (w160:T2)
          n74 = call "fgv_AOL_Globals Write.vi"("AOL_Globals"=w160) -> ()  [unwired: 10 in, 1 out]
          n75 = Unbundle By Name(w151) -> ("XYZ Start"=w153:cluster{"X":sgl, "Y":sgl, "Z":sgl}[])
          n76 = Array Size(array=w153) -> (size(s)=w152:i32)
          n77 = Initialize Array(0.0 ("element"), w152) -> (w149:dbl[])
        }
        frame "Live Volume Imaging" {
          # "Warning!\nThis should always be \"1\" for live imaging. This code needs revising and testing.\nDecide if live plane imaging is to be used."
          # "WARNING!\nUNTESTED!"
          # "Warning!\nReview the code in this case and update it as necessary."
          n78 = Unbundle By Name(w185) -> ("Experiment folder path"=w188:path)
          n79 = call "Experiment header-Save_Load config file data.vi"("Header file actions"=Header_file_actions."Read All", "Header file sections"=Header_file_sections."ALL SECTIONS", "Experiment data folder path"=w188) -> ("All header parameters out"=w187:T13)  [unwired: 7 in, 1 out]
          n80 = Unbundle By Name(w185) -> ("Experiment folder path"=w181:path)
          n81 = Unbundle By Name(w187) -> ("FUNCTIONAL IMAGING.Number of trials"=w184:dbl, "FUNCTIONAL IMAGING.Acquisition Length"=w186:dbl)
          n82 = call "ROI coord bundler.vi"("Experiment folder path"=w181) -> ("Number of POIs"=w173:i32, "ROI Attributes (broken down to miniscans)"=w172:T1[], "Laser(V)"=w171:dbl[], "ROI Coordinates (broken down to miniscans)"=w182:T8, "Total number of miniscans"=w183:i32, "ROI Attributes"=w180:T1[])  [unwired: 8 in, 5 out]
          n83 = To Unsigned Word Integer(number=w173) -> (unsigned 16bit integer=w191:u16)
          n84 = To Unsigned Word Integer(number=w183) -> (unsigned 16bit integer=w190:u16)
          n85 = call "Calculate number of miniscans.vi"("XYZ Coordinates"=w180, "Acquisition length (sec)"=w186) -> ("Number of cycles"=w189:u64, "AOD fill time (us)"=w192:dbl)  [unwired: 7 in, 1 out]
          n86 = Bundle By Name(cluster=w185, "Number of Trials"=w184, "Fill time (us)"=w192, "Number of Cycles"=w189, "Number of POI"=w191, "Number of Miniscans"=w190) -> (w175:T2)
          n87 = call "fgv_AOL_Globals Write.vi"("AOL_Globals"=w175) -> ()  [unwired: 10 in, 1 out]
          n88 = Unbundle By Name(w175) -> ("Number of POI"=w178:u16, "Number of Miniscans"=w179:u16)
          n89 = Equal To 0?(x=w178) -> (x = 0?=w177:bool)
          n90 = Equal To 0?(x=w179) -> (x = 0?=w176:bool)
          n91 = Compound Arithmetic op=AND(w177, w176) -> (w174:bool)
        }
      }
    }
    frame Error {
    }
  }
  "ROI Coordinates (broken down to miniscans)" <- w12
  "error out" <- w10
  "AOL_Globals" <- w4
  "Cycle time (us)" <- w7
  "ROI Attributes (broken down to miniscans)" <- w6
  "Zoom" <- w5
  "NO ROI AVAILABLE!!!" <- w3
  "Laser(V)" <- w1
